vi "test_read-nmea-data2.vi"() -> ()   [LabVIEW 2019] (continued)
F9P\t$GAGSV,2,2,08,12,39,103,,19,25,045,,25,08,248,,36,27,309,,2*70\n\t\n15:14:16.66\tF9P\t$GBGSV,1,1,04,11,48,133,29,14,87,101,29,28,,,29,33,62,220,28,1*4A\n\t\n15:14:16.68\tF9P\t$GBGSV,1,1,03,11,48,133,,14,87,101,,33,62,220,,3*44\n\t\n15:14:16.70\tF9P\t$GNGLL,3723.59237,N,12656.98029,E,061418.00,A,A*7E\n\t\n15:14:16.72\tF9P\t\t\n15:14:16.74\tF9P\t\t\n15:14:16.76\tF9P\t\t\n15:14:16.78\tF9P\t\t\n15:14:16.80\tF9P\t\t\n15:14:16.82\tF9P\t\t\n15:14:16.84\tF9P\t\t\n15:14:16.86\tF9P\t\t\n15:14:16.88\tF9P\t\t\n15:14:16.90\tF9P\t\t\n15:14:16.92\tF9P\t\t\n15:14:16.94\tF9P\t\t\n15:14:16.96\tF9P\t\t\n15:14:16.98\tF9P\t\t\n15:14:17.00\tF9P\t\t\n15:14:17.02\tF9P\t\t\n15:14:17.04\tF9P\t\t\n15:14:17.06\tF9P\t\t\n15:14:17.08\tF9P\t\t\n15:14:17.10\tF9P\t\t\n15:14:17.12\tF9P\t\t\n15:14:17.14\tF9P\t\t\n15:14:17.16\tF9P\t\t\n15:14:17.18\tF9P\t\t\n15:14:17.20\tF9P\t\t\n15:14:17.22\tF9P\t\t\n15:14:17.24\tF9P\t$GNRMC,061419.00,A,3723.59313,N,12656.97992,E,2.358,333.03,250720,,,A,V*0D\n\t\n15:14:17.26\tF9P\t$GNVTG,333.03,T,,M,2.358,N,4.367,K,A*29\n\t\n15:14:17.28\tF9P\t$GNGGA,061419.00,3723.59313,N,12656.97992,E,1,12,0.74,45.0,M,18.5,M,,*76\n\t\n15:14:17.30\tF9P\t$GNGSA,A,3,12,06,19,05,17,09,04,02,,,,,1.28,0.74,1.04,1*0D\n\t\n15:14:17.32\tF9P\t$GNGSA,A,3,85,70,71,84,,,,,,,,,1.28,0.74,1.04,2*0F\n\t\n15:14:17.34\tF9P\t$GNGSA,A,3,36,19,11,04,09,12,,,,,,,1.28,0.74,1.04,3*0D\n\t\n15:14:17.36\tF9P\t$GNGSA,A,3,14,11,33,,,,,,,,,,1.28,0.74,1.04,4*0C\n\t\n15:14:17.38\tF9P\t$GPGSV,3,1,09,02,55,320,28,04,17,043,33,05,38,248,24,06,64,050,30,1*67\n\t\n15:14:17.40\tF9P\t$GPGSV,3,2,09,09,44,073,33,12,23,276,26,17,32,154,38,19,51,157,29,1*6C\n\t\n15:14:17.42\tF9P\t$GPGSV,3,3,09,25,12,306,18,1*55\n\t\n15:14:17.44\tF9P\t$GPGSV,3,1,09,02,55,320,,04,17,043,23,05,38,248,,06,64,050,22,6*6E\n\t\n15:14:17.46\tF9P\t$GPGSV,3,2,09,09,44,073,25,12,23,276,,17,32,154,24,19,51,157,,6*6E\n\t\n15:14:17.48\tF9P\t$GPGSV,3,3,09,25,12,306,,6*5B\n\t\n15:14:17.50\tF9P\t$GLGSV,2,1,08,69,11,031,34,70,70,038,24,71,53,206,39,72,05,210,,1*79\n\t\n15:14:17.52\tF9P\t$GLGSV,2,2,08,77,01,325,,84,19,123,27,85,70,070,38,86,37,330,,1*78\n\t\n15:14:17.54\tF9P\t$GLGSV,2,1,08,69,11,031,27,70,70,038,,71,53,206,28,72,05,210,24,3*79\n\t\n15:14:17.56\tF9P\t$GLGSV,2,2,08,77,01,325,,84,19,123,21,85,70,070,23,86,37,330,,3*76\n\t\n15:14:17.58\tF9P\t$GAGSV,2,1,08,02,08,296,12,04,67,115,30,09,33,193,34,11,72,001,22,7*7E\n\t\n15:14:17.60\tF9P\t$GAGSV,2,2,08,12,39,103,32,19,25,045,28,25,08,248,,36,27,309,11,7*7E\n\t\n15:14:17.62\tF9P\t$GAGSV,2,1,08,02,08,296,,04,67,115,,09,33,193,,11,72,001,,2*7C\n\t\n15:14:17.64\tF9P\t$GAGSV,2,2,08,12,39,103,,19,25,045,,25,08,248,,36,27,309,,2*70\n\t\n15:14:17.66\tF9P\t$GBGSV,1,1,04,11,48,133,29,14,87,101,28,28,,,28,33,62,220,28,1*4A\n\t\n15:14:17.68\tF9P\t$GBGSV,1,1,03,11,48,133,33,14,87,101,,33,62,220,,3*44\n\t\n15:14:17.70\tF9P\t$GNGLL,3723.59313,N,12656.97992,E,061419.00,A,A*7E\n\t\n15:14:17.72\tF9P\t\t\n15:14:17.74\tF9P\t\t\n15:14:17.76\tF9P\t\t\n15:14:17.78\tF9P\t\t\n15:14:17.80\tF9P\t\t\n15:14:17.82\tF9P\t\t\n15:14:17.84\tF9P\t\t\n15:14:17.86\tF9P\t\t\n15:14:17.88\tF9P\t\t\n15:14:17.90\tF9P\t\t\n15:14:17.92\tF9P\t\t\n15:14:17.94\tF9P\t\t\n15:14:17.96\tF9P\t\t\n15:14:17.98\tF9P\t\t\n15:14:18.00\tF9P\t\t\n15:14:18.02\tF9P\t\t\n15:14:18.04\tF9P\t\t\n15:14:18.06\tF9P\t\t\n15:14:18.08\tF9P\t\t\n15:14:18.10\tF9P\t\t\n15:14:18.12\tF9P\t\t\n15:14:18.14\tF9P\t\t\n15:14:18.16\tF9P\t\t\n15:14:18.18\tF9P\t\t\n15:14:18.20\tF9P\t\t\n15:14:18.22\tF9P\t\t\n15:14:18.24\tF9P\t$GNRMC,061420.00,A,3723.59379,N,12656.97968,E,2.022,335.58,250720,,,A,V*08\n\t\n15:14:18.26\tF9P\t$GNVTG,335.58,T,,M,2.022,N,3.745,K,A*2C\n\t\n15:14:18.28\tF9P\t$GNGGA,061420.00,3723.59379,N,12656.97968,E,1,12,0.74,45.1,M,18.5,M,,*74\n\t\n15:14:18.30\tF9P\t$GNGSA,A,3,12,06,19,05,17,09,04,02,,,,,1.28,0.74,1.04,1*0D\n\t\n15:14:18.32\tF9P\t$GNGSA,A,3,85,70,71,84,,,,,,,,,1.28,0.74,1.04,2*0F\n\t\n15:14:18.34\tF9P\t$GNGSA,A,3,36,19,11,04,09,12,,,,,,,1.28,0.74,1.04,3*0D\n\t\n15:14:18.36\tF9P\t$GNGSA,A,3,14,11,33,,,,,,,,,,1.28,0.74,1.04,4*0C\n\t\n15:14:18.38\tF9P\t$GPGSV,3,1,09,02,55,320,27,04,17,043,35,05,38,248,25,06,64,050,30,1*6F\n\t\n15:14:18.40\tF9P\t$GPGSV,3,2,09,09,44,073,28,12,23,276,27,17,32,154,38,19,51,157,39,1*66\n\t\n15:14:18.42\tF9P\t$GPGSV,3,3,09,25,12,306,19,1*54\n\t\n15:14:18.44\tF9P\t$GPGSV,3,1,09,02,55,320,,04,17,043,29,05,38,248,,06,64,050,22,6*64\n\t\n15:14:18.46\tF9P\t$GPGSV,3,2,09,09,44,073,24,12,23,276,,17,32,154,22,19,51,157,,6*69\n\t\n15:14:18.48\tF9P\t$GPGSV,3,3,09,25,12,306,,6*5B\n\t\n15:14:18.50\tF9P\t$GLGSV,2,1,08,69,11,031,37,70,70,038,23,71,53,206,32,72,05,210,,1*76\n\t\n15:14:18.52\tF9P\t$GLGSV,2,2,08,77,01,325,,84,19,123,25,85,70,070,31,86,37,330,,1*73\n\t\n15:14:18.54\tF9P\t$GLGSV,2,1,08,69,11,031,26,70,70,038,,71,53,206,28,72,05,210,20,3*7C\n\t\n15:14:18.56\tF9P\t$GLGSV,2,2,08,77,01,325,,84,19,123,25,85,70,070,22,86,37,330,,3*73\n\t\n15:14:18.58\tF9P\t$GAGSV,2,1,08,02,08,296,10,04,67,115,30,09,33,193,26,11,72,001,23,7*7E\n\t\n15:14:18.60\tF9P\t$GAGSV,2,2,08,12,39,103,27,19,25,045,27,25,08,248,,36,27,309,10,7*74\n\t\n15:14:18.62\tF9P\t$GAGSV,2,1,08,02,08,296,,04,67,115,,09,33,193,,11,72,001,,2*7C\n\t\n15:14:18.64\tF9P\t$GAGSV,2,2,08,12,39,103,,19,25,045,,25,08,248,,36,27,309,,2*70\n\t\n15:14:18.66\tF9P\t$GBGSV,1,1,04,11,48,133,39,14,87,101,28,28,,,32,33,62,220,27,1*4F\n\t\n15:14:18.68\tF9P\t$GBGSV,1,1,03,11,48,133,36,14,87,101,,33,62,220,,3*41\n\t\n15:14:18.70\tF9P\t$GNGLL,3723.59379,N,12656.97968,E,061420.00,A,A*7D\n\t\n15:14:18.72\tF9P\t\t\n15:14:18.74\tF9P\t\t\n15:14:18.76\tF9P\t\t\n15:14:18.78\tF9P\t\t\n15:14:18.80\tF9P\t\t\n15:14:18.82\tF9P\t\t\n15:14:18.84\tF9P\t\t\n15:14:18.86\tF9P\t\t\n15:14:18.88\tF9P\t\t\n15:14:18.90\tF9P\t\t\n15:14:18.92\tF9P\t\t\n15:14:18.94\tF9P\t\t\n15:14:18.96\tF9P\t\t\n15:14:18.98\tF9P\t\t\n15:14:19.00\tF9P\t\t\n15:14:19.02\tF9P\t\t\n15:14:19.04\tF9P\t\t\n15:14:19.06\tF9P\t\t\n15:14:19.08\tF9P\t\t\n15:14:19.10\tF9P\t\t\n15:14:19.12\tF9P\t\t\n15:14:19.14\tF9P\t\t\n15:14:19.16\tF9P\t\t\n15:14:19.18\tF9P\t\t\n15:14:19.20\tF9P\t\t\n15:14:19.22\tF9P\t\t\n15:14:19.24\tF9P\t$GNRMC,061421.00,A,3723.59448,N,12656.98000,E,1.477,359.13,250720,,,A,V*06\n\t\n15:14:19.26\tF9P\t$GNVTG,359.13,T,,M,1.477,N,2.735,K,A*28\n\t\n15:14:19.28\tF9P\t$GNGGA,061421.00,3723.59448,N,12656.98000,E,1,12,0.66,44.4,M,18.5,M,,*7F\n\t\n15:14:19.30\tF9P\t$GNGSA,A,3,12,06,19,05,17,09,04,02,,,,,1.16,0.66,0.95,1*0A\n\t\n15:14:19.32\tF9P\t$GNGSA,A,3,85,70,71,84,,,,,,,,,1.16,0.66,0.95,2*08\n\t\n15:14:19.34\tF9P\t$GNGSA,A,3,36,19,11,04,09,12,,,,,,,1.16,0.66,0.95,3*0A\n\t\n15:14:19.36\tF9P\t$GNGSA,A,3,14,11,33,,,,,,,,,,1.16,0.66,0.95,4*0B\n\t\n15:14:19.38\tF9P\t$GPGSV,3,1,09,02,55,320,27,04,17,043,38,05,38,248,22,06,64,050,34,1*61\n\t\n15:14:19.40\tF9P\t$GPGSV,3,2,09,09,44,073,29,12,23,276,33,17,32,154,38,19,51,157,38,1*63\n\t\n15:14:19.42\tF9P\t$GPGSV,3,3,09,25,12,306,20,1*5E\n\t\n15:14:19.44\tF9P\t$GPGSV,3,1,09,02,55,320,,04,17,043,25,05,38,248,,06,64,050,24,6*6E\n\t\n15:14:19.46\tF9P\t$GPGSV,3,2,09,09,44,073,24,12,23,276,20,17,32,154,21,19,51,157,,6*68\n\t\n15:14:19.49\tF9P\t$GPGSV,3,3,09,25,12,306,,6*5B\n\t\n15:14:19.51\tF9P\t$GLGSV,2,1,08,69,11,031,40,70,70,038,24,71,53,206,32,72,05,210,,1*71\n\t\n15:14:19.53\tF9P\t$GLGSV,2,2,08,77,01,325,,84,19,123,24,85,70,070,32,86,37,330,,1*71\n\t\n15:14:19.55\tF9P\t$GLGSV,2,1,08,69,11,031,28,70,70,038,,71,53,206,26,72,05,210,,3*7E\n\t\n15:14:19.57\tF9P\t$GLGSV,2,2,08,77,01,325,,84,19,123,24,85,70,070,21,86,37,330,,3*71\n\t\n15:14:19.59\tF9P\t$GAGSV,2,1,08,02,08,296,07,04,67,115,28,09,33,193,31,11,72,001,24,7*70\n\t\n15:14:19.61\tF9P\t$GAGSV,2,2,08,12,39,103,27,19,25,045,31,25,08,248,,36,27,309,12,7*71\n\t\n15:14:19.63\tF9P\t$GAGSV,2,1,08,02,08,296,,04,67,115,,09,33,193,,11,72,001,,2*7C\n\t\n15:14:19.65\tF9P\t$GAGSV,2,2,08,12,39,103,,19,25,045,,25,08,248,,36,27,309,,2*70\n\t\n15:14:19.67\tF9P\t$GBGSV,1,1,04,11,48,133,37,14,87,101,28,28,,,27,33,62,220,26,1*44\n\t\n15:14:19.69\tF9P\t$GBGSV,1,1,03,11,48,133,28,14,87,101,,33,62,220,,3*4E\n\t\n15:14:19.71\tF9P\t$GNGLL,3723.59448,N,12656.98000,E,061421.00,A,A*71\n\t\n15:14:19.73\tF9P\t\t\n15:14:19.75\tF9P\t\t\n15:14:19.77\tF9P\t\t\n15:14:19.79\tF9P\t\t\n15:14:19.81\tF9P\t\t\n15:14:19.83\tF9P\t\t\n15:14:19.85\tF9P\t\t\n15:14:19.87\tF9P\t\t\n15:14:19.89\tF9P\t\t\n15:14:19.91\tF9P\t\t\n15:14:19.93\tF9P\t\t\n15:14:19.95\tF9P\t\t\n15:14:19.97\tF9P\t\t\n15:14:19.99\tF9P\t\t\n15:14:20.01\tF9P\t\t\n15:14:20.03\tF9P\t\t\n15:14:20.05\tF9P\t\t\n15:14:20.07\tF9P\t\t\n15:14:20.09\tF9P\t\t\n15:14:20.11\tF9P\t\t\n15:14:20.13\tF9P\t\t\n15:14:20.15\tF9P\t\t\n15:14:20.17\tF9P\t\t\n15:14:20.19\tF9P\t\t\n15:14:20.21\tF9P\t\t\n15:14:20.23\tF9P\t\t\n15:14:20.25\tF9P\t$GNRMC,061422.00,A,3723.59517,N,12656.97994,E,2.094,356.24,250720,,,A,V*04\n\t\n15:14:20.27\tF9P\t$GNVTG,356.24,T,,M,2.094,N,3.877,K,A*21\n\t\n15:14:20.29\tF9P\t$GNGGA,061422.00,3723.59517,N,12656.97994,E,1,12,0.66,44.6,M,18.5,M,,*7E\n\t\n15:14:20.31\tF9P\t$GNGSA,A,3,12,06,19,05,17,09,04,02,,,,,1.16,0.66,0.95,1*0A\n\t\n15:14:20.33\tF9P\t$GNGSA,A,3,85,70,71,84,,,,,,,,,1.16,0.66,0.95,2*08\n\t\n15:14:20.35\tF9P\t$GNGSA,A,3,36,19,11,04,09,12,,,,,,,1.16,0.66,0.95,3*0A\n\t\n15:14:20.37\tF9P\t$GNGSA,A,3,14,11,33,,,,,,,,,,1.16,0.66,0.95,4*0B\n\t\n15:14:20.39\tF9P\t$GPGSV,3,1,09,02,55,320,31,04,17,043,31,05,38,248,29,06,64,050,29,1*68\n\t\n15:14:20.41\tF9P\t$GPGSV,3,2,09,09,44,073,36,12,23,276,27,17,32,154,31,19,51,157,40,1*6E\n\t\n15:14:20.43\tF9P\t$GPGSV,3,3,09,25,12,306,21,1*5F\n\t\n15:14:20.45\tF9P\t$GPGSV,3,1,09,02,55,320,,04,17,043,26,05,38,248,,06,64,050,25,6*6C\n\t\n15:14:20.47\tF9P\t$GPGSV,3,2,09,09,44,073,26,12,23,276,18,17,32,154,21,19,51,157,,6*61\n\t\n15:14:20.49\tF9P\t$GPGSV,3,3,09,25,12,306,,6*5B\n\t\n15:14:20.51\tF9P\t$GLGSV,2,1,08,69,11,031,30,70,70,038,25,71,53,206,26,72,05,210,,1*72\n\t\n15:14:20.53\tF9P\t$GLGSV,2,2,08,77,01,325,,84,19,123,20,85,70,070,35,86,37,330,,1*72\n\t\n15:14:20.55\tF9P\t$GLGSV,2,1,08,69,11,031,26,70,70,038,,71,53,206,23,72,05,210,,3*75\n\t\n15:14:20.57\tF9P\t$GLGSV,2,2,08,77,01,325,,84,19,123,24,85,70,070,22,86,37,330,,3*72\n\t\n15:14:20.59\tF9P\t$GAGSV,2,1,08,02,08,296,10,04,67,115,28,09,33,193,34,11,72,001,24,7*73\n\t\n15:14:20.61\tF9P\t$GAGSV,2,2,08,12,39,103,30,19,25,045,27,25,08,248,,36,27,309,14,7*76\n\t\n15:14:20.63\tF9P\t$GAGSV,2,1,08,02,08,296,,04,67,115,,09,33,193,,11,72,001,,2*7C\n\t\n15:14:20.65\tF9P\t$GAGSV,2,2,08,12,39,103,,19,25,045,,25,08,248,,36,27,309,,2*70\n\t\n15:14:20.67\tF9P\t$GBGSV,1,1,04,11,48,133,26,14,87,101,28,28,,,31,33,62,220,25,1*40\n\t\n15:14:20.69\tF9P\t$GBGSV,1,1,03,11,48,133,27,14,87,101,,33,62,220,,3*41\n\t\n15:14:20.71\tF9P\t$GNGLL,3723.59517,N,12656.97994,E,061422.00,A,A*72\n\t\n15:14:20.73\tF9P\t\t\n15:14:20.75\tF9P\t\t\n15:14:20.77\tF9P\t\t\n15:14:20.79\tF9P\t\t\n15:14:20.81\tF9P\t\t\n15:14:20.83\tF9P\t\t\n15:14:20.85\tF9P\t\t\n15:14:20.87\tF9P\t\t\n15:14:20.89\tF9P\t\t\n15:14:20.91\tF9P\t\t\n15:14:20.93\tF9P\t\t\n15:14:20.95\tF9P\t\t\n15:14:20.97\tF9P\t\t\n15:14:20.99\tF9P\t\t\n15:14:21.01\tF9P\t\t\n15:14:21.03\tF9P\t\t\n15:14:21.05\tF9P\t\t\n15:14:21.07\tF9P\t\t\n15:14:21.09\tF9P\t\t\n15:14:21.11\tF9P\t\t\n15:14:21.13\tF9P\t\t\n15:14:21.15\tF9P\t\t\n15:14:21.17\tF9P\t\t\n15:14:21.19\tF9P\t\t\n15:14:21.21\tF9P\t\t\n15:14:21.23\tF9P\t\t\n15:14:21.25\tF9P\t$GNRMC,061423.00,A,3723.59599,N,12656.97945,E,2.578,336.99,250720,,,A,V*08\n\t\n15:14:21.27\tF9P\t$GNVTG,336.99,T,,M,2.578,N,4.775,K,A*2C\n\t\n15:14:21.29\tF9P\t$GNGGA,061423.00,3723.59599,N,12656.97945,E,1,12,0.63,44.6,M,18.5,M,,*70\n\t\n15:14:21.31\tF9P\t$GNGSA,A,3,12,06,19,05,17,09,04,02,,,,,1.14,0.63,0.95,1*0D\n\t\n15:14:21.33\tF9P\t$GNGSA,A,3,85,70,71,84,,,,,,,,,1.14,0.63,0.95,2*0F\n\t\n15:14:21.35\tF9P\t$GNGSA,A,3,36,19,11,04,09,12,,,,,,,1.14,0.63,0.95,3*0D\n\t\n15:14:21.37\tF9P\t$GNGSA,A,3,14,11,33,,,,,,,,,,1.14,0.63,0.95,4*0C\n\t\n15:14:21.39\tF9P\t$GPGSV,3,1,09,02,55,320,26,04,17,043,29,05,38,248,30,06,64,050,29,1*6F\n\t\n15:14:21.41\tF9P\t$GPGSV,3,2,09,09,44,073,33,12,23,276,26,17,32,154,33,19,51,157,28,1*66\n\t\n15:14:21.43\tF9P\t$GPGSV,3,3,09,25,12,306,21,1*5F\n\t\n15:14:21.45\tF9P\t$GPGSV,3,1,09,02,55,320,,04,17,043,26,05,38,248,,06,64,050,25,6*6C\n\t\n15:14:21.47\tF9P\t$GPGSV,3,2,09,09,44,073,25,12,23,276,17,17,32,154,20,19,51,157,,6*6C\n\t\n15:14:21.49\tF9P\t$GPGSV,3,3,09,25,12,306,,6*5B\n\t\n15:14:21.51\tF9P\t$GLGSV,2,1,08,69,11,031,37,70,70,038,26,71,53,206,26,72,05,210,,1*76\n\t\n15:14:21.53\tF9P\t$GLGSV,2,2,08,77,01,325,,84,19,123,20,85,70,070,37,86,37,330,,1*70\n\t\n15:14:21.55\tF9P\t$GLGSV,2,1,08,69,11,031,26,70,70,038,,71,53,206,19,72,05,210,,3*7C\n\t\n15:14:21.57\tF9P\t$GLGSV,2,2,08,77,01,325,,84,19,123,24,85,70,070,23,86,37,330,,3*73\n\t\n15:14:21.59\tF9P\t$GAGSV,2,1,08,02,08,296,10,04,67,115,34,09,33,193,31,11,72,001,24,7*7B\n\t\n15:14:21.61\tF9P\t$GAGSV,2,2,08,12,39,103,29,19,25,045,26,25,08,248,,36,27,309,13,7*78\n\t\n15:14:21.63\tF9P\t$GAGSV,2,1,08,02,08,296,,04,67,115,,09,33,193,,11,72,001,,2*7C\n\t\n15:14:21.65\tF9P\t$GAGSV,2,2,08,12,39,103,,19,25,045,,25,08,248,,36,27,309,,2*70\n\t\n15:14:21.67\tF9P\t$GBGSV,2,1,05,07,,,30,11,48,133,27,14,87,101,35,28,,,26,1*7E\n\t\n15:14:21.69\tF9P\t$GBGSV,2,2,05,33,62,220,24,1*41\n\t\n15:14:21.71\tF9P\t$GBGSV,1,1,03,11,48,133,,14,87,101,,33,62,220,,3*44\n\t\n15:14:21.73\tF9P\t$GNGLL,3723.59599,N,12656.97945,E,061423.00,A,A*79\n\t\n15:14:21.75\tF9P\t\t\n15:14:21.77\tF9P\t\t\n15:14:21.79\tF9P\t\t\n15:14:21.81\tF9P\t\t\n15:14:21.83\tF9P\t\t\n15:14:21.85\tF9P\t\t\n15:14:21.87\tF9P\t\t\n15:14:21.89\tF9P\t\t\n15:14:21.91\tF9P\t\t\n15:14:21.93\tF9P\t\t\n15:14:21.95\tF9P\t\t\n15:14:21.97\tF9P\t\t\n15:14:21.99\tF9P\t\t\n15:14:22.01\tF9P\t\t\n15:14:22.03\tF9P\t\t\n15:14:22.05\tF9P\t\t\n15:14:22.07\tF9P\t\t\n15:14:22.09\tF9P\t\t\n15:14:22.11\tF9P\t\t\n15:14:22.13\tF9P\t\t\n15:14:22.15\tF9P\t\t\n15:14:22.17\tF9P\t\t\n15:14:22.19\tF9P\t\t\n15:14:22.21\tF9P\t\t\n15:14:22.23\tF9P\t$GNRMC,061424.00,A,3723.59662,N,12656.97913,E,2.085,332.88,250720,,,A,V*08\n\t\n15:14:22.25\tF9P\t$GNVTG,332.88,T,,M,2.085,N,3.861,K,A*22\n\t\n15:14:22.27\tF9P\t$GNGGA,061424.00,3723.59662,N,12656.97913,E,1,12,0.66,44.6,M,18.5,M,,*76\n\t\n15:14:22.29\tF9P\t$GNGSA,A,3,12,06,19,05,17,09,04,02,,,,,1.17,0.66,0.97,1*09\n\t\n15:14:22.31\tF9P\t$GNGSA,A,3,85,70,71,84,,,,,,,,,1.17,0.66,0.97,2*0B\n\t\n15:14:22.33\tF9P\t$GNGSA,A,3,36,19,11,04,09,12,,,,,,,1.17,0.66,0.97,3*09\n\t\n15:14:22.35\tF9P\t$GNGSA,A,3,14,11,33,,,,,,,,,,1.17,0.66,0.97,4*08\n\t\n15:14:22.37\tF9P\t$GPGSV,3,1,09,02,55,320,28,04,17,043,33,05,38,248,33,06,64,050,29,1*69\n\t\n15:14:22.39\tF9P\t$GPGSV,3,2,09,09,44,073,32,12,23,276,26,17,32,154,39,19,51,157,32,1*66\n\t\n15:14:22.41\tF9P\t$GPGSV,3,3,09,25,12,306,22,1*5C\n\t\n15:14:22.43\tF9P\t$GPGSV,3,1,09,02,55,320,,04,17,043,25,05,38,248,,06,64,050,24,6*6E\n\t\n15:14:22.45\tF9P\t$GPGSV,3,2,09,09,44,073,25,12,23,276,16,17,32,154,22,19,51,157,,6*6F\n\t\n15:14:22.47\tF9P\t$GPGSV,3,3,09,25,12,306,,6*5B\n\t\n15:14:22.49\tF9P\t$GLGSV,2,1,08,69,10,031,35,70,70,038,25,71,53,206,26,72,05,210,,1*76\n\t\n15:14:22.51\tF9P\t$GLGSV,2,2,08,77,01,325,,84,19,123,19,85,70,070,34,86,37,330,,1*79\n\t\n15:14:22.53\tF9P\t$GLGSV,2,1,08,69,10,031,27,70,70,038,,71,53,206,17,72,05,210,,3*72\n\t\n15:14:22.55\tF9P\t$GLGSV,2,2,08,77,01,325,,84,19,123,24,85,70,070,24,86,37,330,,3*74\n\t\n15:14:22.57\tF9P\t$GAGSV,2,1,08,02,08,296,09,04,67,115,30,09,33,193,24,11,72,001,23,7*74\n\t\n15:14:22.59\tF9P\t$GAGSV,2,2,08,12,39,103,36,19,25,045,28,25,08,248,,36,27,309,16,7*7D\n\t\n15:14:22.61\tF9P\t$GAGSV,2,1,08,02,08,296,,04,67,115,,09,33,193,,11,72,001,,2*7C\n\t\n15:14:22.63\tF9P\t$GAGSV,2,2,08,12,39,103,,19,25,045,,25,08,248,,36,27,309,,2*70\n\t\n15:14:22.65\tF9P\t$GBGSV,2,1,05,07,,,30,11,48,133,26,14,87,101,29,28,,,27,1*73\n\t\n15:14:22.67\tF9P\t$GBGSV,2,2,05,33,62,220,23,1*46\n\t\n15:14:22.69\tF9P\t$GBGSV,1,1,03,11,48,133,,14,87,101,,33,62,220,,3*44\n\t\n15:14:22.71\tF9P\t$GNGLL,3723.59662,N,12656.97913,E,061424.00,A,A*7A\n\t\n15:14:22.73\tF9P\t\t\n15:14:22.75\tF9P\t\t\n15:14:22.77\tF9P\t\t\n15:14:22.79\tF9P\t\t\n15:14:22.81\tF9P\t\t\n15:14:22.83\tF9P\t\t\n15:14:22.85\tF9P\t\t\n15:14:22.87\tF9P\t\t\n15:14:22.89\tF9P\t\t\n15:14:22.91\tF9P\t\t\n15:14:22.93\tF9P\t\t\n15:14:22.95\tF9P\t\t\n15:14:22.97\tF9P\t\t\n15:14:22.99\tF9P\t\t\n15:14:23.01\tF9P\t\t\n15:14:23.03\tF9P\t\t\n15:14:23.05\tF9P\t\t\n15:14:23.07\tF9P\t\t\n15:14:23.09\tF9P\t\t\n15:14:23.11\tF9P\t\t\n15:14:23.13\tF9P\t\t\n15:14:23.15\tF9P\t\t\n15:14:23.17\tF9P\t\t\n15:14:23.19\tF9P\t\t\n15:14:23.21\tF9P\t\t\n15:14:23.23\tF9P\t$GNRMC,061425.00,A,3723.59727,N,12656.97873,E,2.179,332.41,250720,,,A,V*09\n\t\n15:14:23.25\tF9P\t$GNVTG,332.41,T,,M,2.179,N,4.036,K,A*28\n\t\n15:14:23.27\tF9P\t$GNGGA,061425.00,3723.59727,N,12656.97873,E,1,12,0.66,44.7,M,18.5,M,,*71\n\t\n15:14:23.29\tF9P\t$GNGSA,A,3,12,06,19,05,17,09,04,02,,,,,1.17,0.66,0.97,1*09\n\t\n15:14:23.31\tF9P\t$GNGSA,A,3,85,70,71,84,,,,,,,,,1.17,0.66,0.97,2*0B\n\t\n15:14:23.33\tF9P\t$GNGSA,A,3,36,19,11,04,09,12,,,,,,,1.17,0.66,0.97,3*09\n\t\n15:14:23.35\tF9P\t$GNGSA,A,3,14,11,33,,,,,,,,,,1.17,0.66,0.97,4*08\n\t\n15:14:23.37\tF9P\t$GPGSV,3,1,09,02,55,320,32,04,17,043,29,05,38,248,41,06,64,050,28,1*6D\n\t\n15:14:23.39\tF9P\t$GPGSV,3,2,09,09,44,073,30,12,23,276,24,17,32,154,42,19,51,157,31,1*69\n\t\n15:14:23.41\tF9P\t$GPGSV,3,3,09,25,12,306,25,1*5B\n\t\n15:14:23.43\tF9P\t$GPGSV,3,1,09,02,55,320,,04,17,043,25,05,38,248,,06,64,050,23,6*69\n\t\n15:14:23.45\tF9P\t$GPGSV,3,2,09,09,44,073,25,12,23,276,14,17,32,154,25,19,51,157,,6*6A\n\t\n15:14:23.47\tF9P\t$GPGSV,3,3,09,25,12,306,,6*5B\n\t\n15:14:23.49\tF9P\t$GLGSV,2,1,08,69,10,031,38,70,70,037,24,71,53,206,25,72,05,210,,1*76\n\t\n15:14:23.51\tF9P\t$GLGSV,2,2,08,77,01,325,,84,19,123,20,85,70,070,32,86,37,330,,1*75\n\t\n15:14:23.53\tF9P\t$GLGSV,2,1,08,69,10,031,28,70,70,037,,71,53,206,15,72,05,210,,3*70\n\t\n15:14:23.55\tF9P\t$GLGSV,2,2,08,77,01,325,,84,19,123,22,85,70,070,23,86,37,330,,3*75\n\t\n15:14:23.57\tF9P\t$GAGSV,2,1,08,02,08,296,09,04,67,115,32,09,33,193,30,11,72,001,23,7*73\n\t\n15:14:23.59\tF9P\t$GAGSV,2,2,08,12,39,103,34,19,25,045,27,25,08,248,,36,27,309,16,7*70\n\t\n15:14:23.61\tF9P\t$GAGSV,2,1,08,02,08,296,,04,67,115,,09,33,193,,11,72,001,23,2*7D\n\t\n15:14:23.63\tF9P\t$GAGSV,2,2,08,12,39,103,28,19,25,045,,25,08,248,,36,27,309,,2*7A\n\t\n15:14:23.65\tF9P\t$GBGSV,2,1,05,07,,,32,11,48,133,34,14,87,101,30,28,,,27,1*7A\n\t\n15:14:23.67\tF9P\t$GBGSV,2,2,05,33,62,220,23,1*46\n\t\n15:14:23.69\tF9P\t$GBGSV,1,1,03,11,48,133,,14,87,101,28,33,62,220,,3*4E\n\t\n15:14:23.71\tF9P\t$GNGLL,3723.59727,N,12656.97873,E,061425.00,A,A*7C\n\t\n15:14:23.73\tF9P\t\t\n15:14:23.75\tF9P\t\t\n15:14:23.77\tF9P\t\t\n15:14:23.79\tF9P\t\t\n15:14:23.81\tF9P\t\t\n15:14:23.83\tF9P\t\t\n15:14:23.85\tF9P\t\t\n15:14:23.87\tF9P\t\t\n15:14:23.89\tF9P\t\t\n15:14:23.91\tF9P\t\t\n15:14:23.93\tF9P\t\t\n15:14:23.95\tF9P\t\t\n15:14:23.97\tF9P\t\t\n15:14:23.99\tF9P\t\t\n15:14:24.01\tF9P\t\t\n15:14:24.03\tF9P\t\t\n15:14:24.05\tF9P\t\t\n15:14:24.07\tF9P\t\t\n15:14:24.09\tF9P\t\t\n15:14:24.11\tF9P\t\t\n15:14:24.13\tF9P\t\t\n15:14:24.15\tF9P\t\t\n15:14:24.17\tF9P\t\t\n15:14:24.19\tF9P\t\t\n15:14:24.21\tF9P\t\t\n15:14:24.23\tF9P\t$GNRMC,061426.00,A,3723.59802,N,12656.97828,E,2.089,333.13,250720,,,A,V*04\n\t\n15:14:24.25\tF9P\t$GNVTG,333.13,T,,M,2.089,N,3.869,K,A*25\n\t\n15:14:24.27\tF9P\t$GNGGA,061426.00,3723.59802,N,12656.97828,E,1,12,0.63,44.1,M,18.5,M,,*77\n\t\n15:14:24.29\tF9P\t$GNGSA,A,3,12,06,19,05,17,09,04,02,,,,,1.14,0.63,0.95,1*0D\n\t\n15:14:24.31\tF9P\t$GNGSA,A,3,85,70,71,84,,,,,,,,,1.14,0.63,0.95,2*0F\n\t\n15:14:24.33\tF9P\t$GNGSA,A,3,36,19,11,04,09,12,,,,,,,1.14,0.63,0.95,3*0D\n\t\n15:14:24.35\tF9P\t$GNGSA,A,3,14,11,33,,,,,,,,,,1.14,0.63,0.95,4*0C\n\t\n15:14:24.37\tF9P\t$GPGSV,3,1,09,02,55,320,32,04,17,043,34,05,38,248,36,06,64,050,28,1*61\n\t\n15:14:24.39\tF9P\t$GPGSV,3,2,09,09,44,073,34,12,23,276,25,17,32,154,35,19,51,157,31,1*6C\n\t\n15:14:24.41\tF9P\t$GPGSV,3,3,09,25,12,306,22,1*5C\n\t\n15:14:24.43\tF9P\t$GPGSV,3,1,09,02,55,320,,04,17,043,24,05,38,248,23,06,64,050,24,6*6E\n\t\n15:14:24.45\tF9P\t$GPGSV,3,2,09,09,44,073,26,12,23,276,14,17,32,154,24,19,51,157,,6*68\n\t\n15:14:24.47\tF9P\t$GPGSV,3,3,09,25,12,306,,6*5B\n\t
